vi "Init.vi"() -> ()   [LabVIEW 2019]
uses:
  D:/SOFT_REPO_GUM/renishawxl80sdk/Dllx64/ComDX10Adaptor.dll
  SOFT_REPO_GUM/renishawxl80sdk/Dllx64/ComDX10Adaptor.dll
panel:
  out "value__":i32
  out "StraightnessShort":i32(ring) items=["None", "LinearPlane", "LinearRetro", "Angular", "StraightnessShort", "StraightnessLong", "VelocityRetro"]
  out "StraightnessLong":i32(ring) items=["None", "LinearPlane", "LinearRetro", "Angular", "StraightnessShort", "StraightnessLong", "VelocityRetro"]
  out "None":i32(ring) items=["None", "LinearPlane", "LinearRetro", "Angular", "StraightnessShort", "StraightnessLong", "VelocityRetro"]
  out "LinearRetro":i32(ring) items=["None", "LinearPlane", "LinearRetro", "Angular", "StraightnessShort", "StraightnessLong", "VelocityRetro"]
  out "LinearPlane":i32(ring) items=["None", "LinearPlane", "LinearRetro", "Angular", "StraightnessShort", "StraightnessLong", "VelocityRetro"]
  out "Angular":i32(ring) items=["None", "LinearPlane", "LinearRetro", "Angular", "StraightnessShort", "StraightnessLong", "VelocityRetro"]
  out "reference out":refnum<k24>
  out "error out 3":errorcluster
  out "XL10Version":string
  out "XL10Status":i32(ring) items=["None"=0, "AveragingOn"=1, "TPInSelected"=4, "BeamLow"=64, "BeamLoss"=128, "StabilityLoss"=256, "Preheat"=2048, "LaserTooCold"=4096, "LaserTooHot"=8192, "LaserUnstable"=16384, "LaserFail"=32768, "NotResponding"=65536, "LongTermAveragingOn"=524288, "MeasurementMode"=7340032, "HighSpeedError"=8388608, "DynamicSelected"=16777216]
  out "SignalStrength":dbl
  out "SerialNumber":string
  out "OpticsFactor":dbl
  out "MeasurementMode":i32(ring) items=["None", "LinearPlane", "LinearRetro", "Angular", "StraightnessShort", "StraightnessLong", "VelocityRetro"]
  out "IsConnected":bool
  out "error out 2":errorcluster
  out "error out":errorcluster
  out "ConnectionString":string
  out "XC10Version":string
  out "XC10Status":i32(ring) items=["Connected"=0, "NotResponding"=65536]
  in  ".NET Container":refnum<k24>(container)
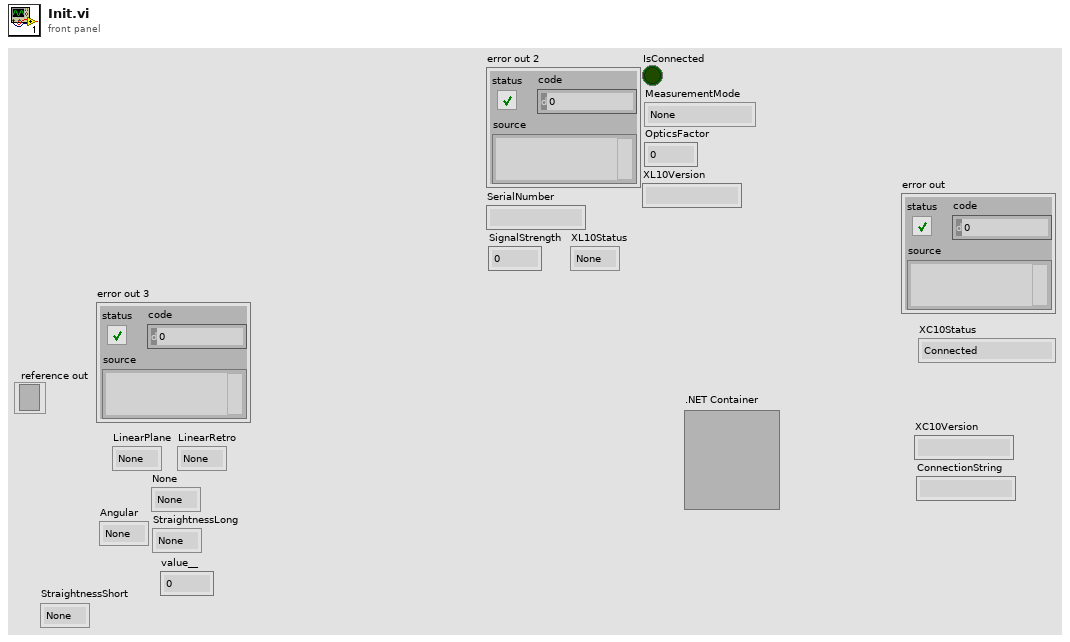
[diagram p1: front panel]
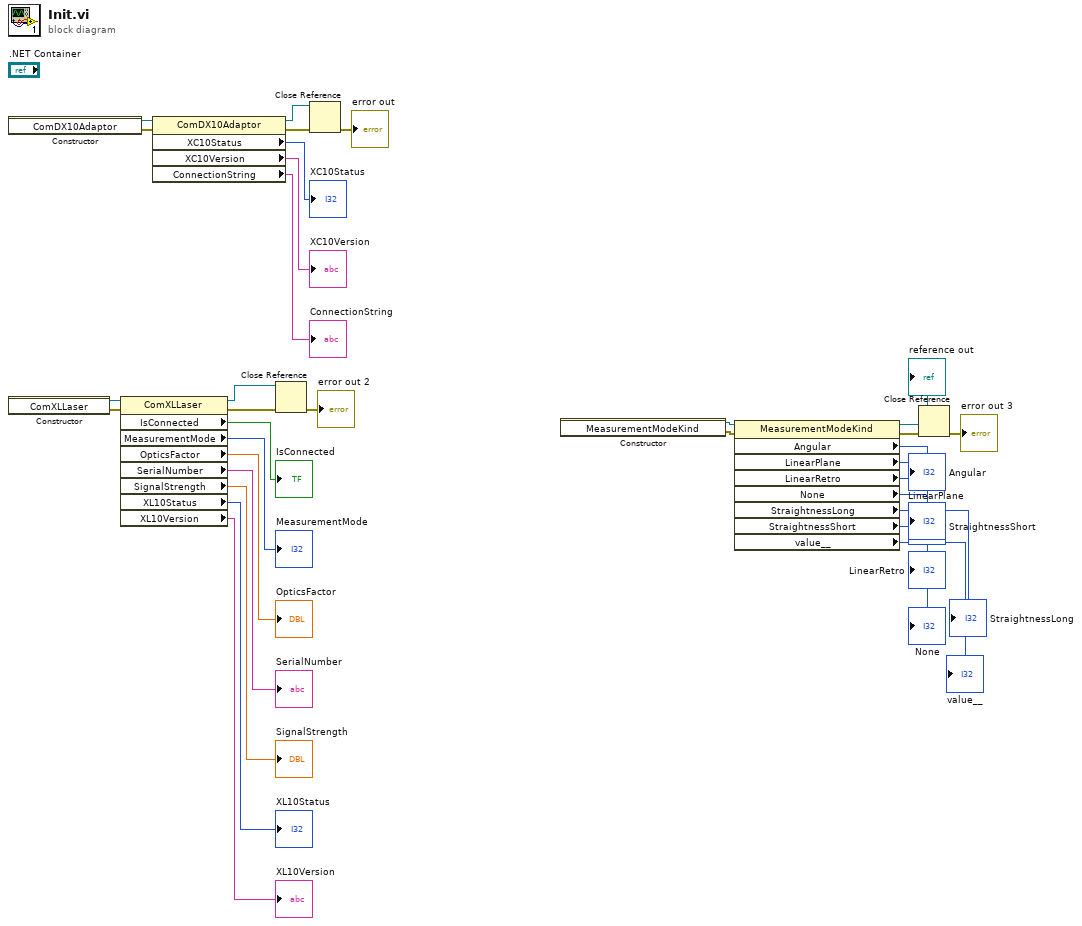
[diagram p0: block diagram]
diagram:
  n1 = constructor class="ComDX10Adaptor"() -> (reference out=w32:refnum<k24>, error out=w25:errorcluster)  [unwired: 3 in, 1 out]
  n2 = constructor class="ComXLLaser"() -> (reference out=w23:refnum<k24>, error out=w24:errorcluster)  [unwired: 3 in, 1 out]
  n3 = property class="ComXLLaser"(reference=w23, error in=w24) -> (reference out=w22:refnum<k24>, error out=w21:errorcluster, "IsConnected"=→"IsConnected":bool, "MeasurementMode"=→"MeasurementMode":i32, "OpticsFactor"=→"OpticsFactor":dbl, "SerialNumber"=→"SerialNumber":string, "SignalStrength"=→"SignalStrength":dbl, "XL10Status"=→"XL10Status":i32, "XL10Version"=→"XL10Version":string)
  n4 = property class="ComDX10Adaptor"(reference=w32, error in=w25) -> (reference out=w28:refnum<k24>, error out=w27:errorcluster, "XC10Status"=→"XC10Status":i32, "XC10Version"=→"XC10Version":string, "ConnectionString"=→"ConnectionString":string)
  n5 = Close Reference(reference=w22, error in (no error)=w21) -> (error out=→"error out 2":errorcluster)
  n6 = Close Reference(reference=w28, error in (no error)=w27) -> (error out=→"error out":errorcluster)
  n7 = constructor class="MeasurementModeKind"() -> (reference out=w10:refnum<k24>, error out=w9:errorcluster)  [unwired: 3 in, 1 out]
  n8 = property class="MeasurementModeKind"(reference=w10, error in=w9) -> (reference out=→"reference out":refnum<k24>, error out=w11:errorcluster, "Angular"=→"Angular":i32, "LinearPlane"=→"LinearPlane":i32, "LinearRetro"=→"LinearRetro":i32, "None"=→"None":i32, "StraightnessLong"=→"StraightnessLong":i32, "StraightnessShort"=→"StraightnessShort":i32, "value__"=→"value__":i32)
  n9 = Close Reference(error in (no error)=w11) -> (error out=→"error out 3":errorcluster)  [unwired: 1 in]
